vi "Excel Write Headers.vi"(8 "Error In":errorcluster, 10 "Header Info":string[](array[string]), 11 "Sheets Ref In":refnum<k7>) -> (0 "Error Out":errorcluster, 3 "Sheets Ref Out":refnum<k7>)   [LabVIEW 2013]
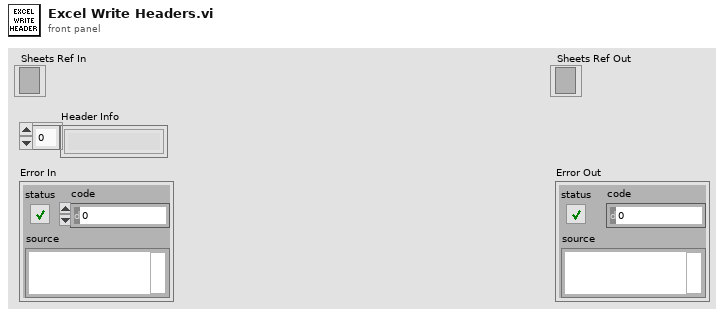
[diagram p1: front panel]
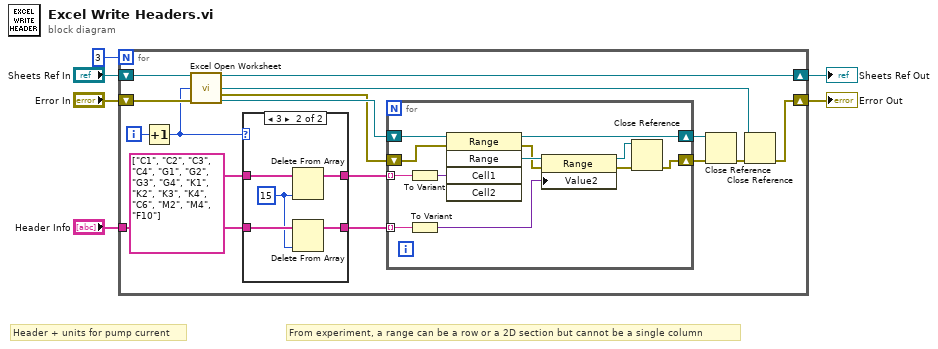
[diagram p0: block diagram]
diagram:
  # "Header + units for pump current"
  # "From experiment, a range can be a row or a 2D section but cannot be a single column"
  n1 = for {
    N: 3 -> [_]
    shift-right: [w19] -> w2
    shift-left: "Error In" -> [w17]
    shift-right: [w15] -> w5
    shift-left: "Sheets Ref In" -> [w16]
    tunnel: "Header Info" -> [w10]
    i -> [w18]
    n2 = Increment(x=w18) -> (x+1=w11:i32)
    n3 = call "Excel Open Worksheet.vi"("Sheets Ref In"=w16, "Sheet#"=w11, "Error In"=w17) -> ("Sheets Ref Out"=w15:refnum<k7>, "Worksheet Ref Out"=w12:refnum<k7>, "Error Out"=w13:errorcluster, "Cells Ref Out"=w14:refnum<k7>)  [unwired: 9 in]
    n4 = case shown="3" w11 {
      tunnel: w10 -> [w23 w29]
      tunnel: [w24 w27] -> w9
      tunnel: string[] ["C1", "C2", "C3", "C4", "G1", "G2", "G3", "G4", "K1", "K2", "K3", "K4", "C6", "M2", "M4", "F10"] -> [w24 w26]
      tunnel: [w23 w28] -> w7
      frame Default {
      }
      frame 3 {
        w25 = 15 ("index")
        n5 = Delete From Array(array=w26, index=w25) -> (array with subset deleted=w27:string[])  [unwired: 1 in, 1 out]
        n6 = Delete From Array(array=w29, index=w25) -> (array with subset deleted=w28:string[])  [unwired: 1 in, 1 out]
      }
    }
    n7 = for {
      shift-right: [w36] -> w20
      shift-left: w13 -> [w41]
      shift-right: [w35] -> w21
      shift-left: w14 -> [w34]
      tunnel: w7 -> [w33] mode=indexing
      tunnel: w9 -> [w32] mode=indexing
      n8 = To Variant(anything=w32) -> (Variant=w39:variant)
      n9 = To Variant(anything=w33) -> (Variant=w37:variant)
      n10 = invoke class="Range" method="Range"(reference=w34, error in=w41, "Cell1"=w39) -> (reference out=w35:refnum<k7>, error out=w38:errorcluster, "Range"=w40:refnum<k7>)  [unwired: 2 in, 2 out]
      n11 = property class="Range"(reference=w40, error in=w38, "Value2"=w37) -> (reference out=w31:refnum<k7>, error out=w30:errorcluster)
      n12 = Close Reference(reference=w31, error in (no error)=w30) -> (error out=w36:errorcluster)
    }
    n13 = Close Reference(reference=w21, error in (no error)=w20) -> (error out=w22:errorcluster)
    n14 = Close Reference(reference=w12, error in (no error)=w22) -> (error out=w19:errorcluster)
  }
  "Sheets Ref Out" <- w5
  "Error Out" <- w2
